vi "Save sxm File.vi"(4 "Parameters":string[][](array[string]), 5 "Auto file naming? (T)":bool=TRUE, 6 "Scanfield":T1, 7 "Scan param":T2, 8 "error in (no error)":errorcluster, 9 "Channels data":cluster{"Forward":sgl[][], "Backward":sgl[][]}[](array[cluster]), 10 "Channels config":T3(array[cluster]), 11 "Filename control":cluster{"Path":path, "Basename":string}={"Path"=path "C:/", "Basename"="unnamed"}) -> (0 "error out":errorcluster, 2 "File path out":path, 3 "Filename control out":cluster{"Path":path, "Basename":string}={"Path"=path "C:/", "Basename"="unnamed"})   [LabVIEW 2016, in "Nanonis Prog Interface.lvlib"]
doc: "<b>Saves a .sxm file.</b>\n\nIt saves the attributes in the header, and the channels configuration and their corresponding data into a .sxm file.\n\n<B>Auto file naming?</B>: if True (default), the file names are \"basenameNNN.sxm\" where NNN is an automatically increasing number.\n<B>Scan param</B>: scan direction Up (True) or Down (False), scan speed in seconds per line, start time, and end time.\n<B>Filename control</B>: the .sxm file is defined through a base path and a base name.\n<B>Channels config</B>: array of channels to save. Contains the channel name, calibration, offset, and channel index.\n<B>Channels data</B>: array of clusters containing forward and backward data for every channel.\n<B>Scanfield</B>: dimension of the scan field (center X & center Y, angle, width & height) and scan resolution (pixels & lines).\n<B>Parameters</B>: rest of header information. The first column should be filled in with the parameter name, and the second column with the parameter value.\nThe Bias value can be inserted using \"BIAS\" or \"Bias (V)\" as the parameter name. If no parameter with the latter name is found in the parameters array, then the file header will show a line as follows:\n:BIAS: n/a\n<B>File path out</B>: returns the full path of the saved fle.\n\nSeveral functions in the Scan palette (like ScanBuffer Get, ScanFrame Get, and Scan Grab Frame Data) can be used to feed in the required information from above.\n\n- Nanonis Programming Interface -"
uses:
  Nanonis Prog Interface.lvlib
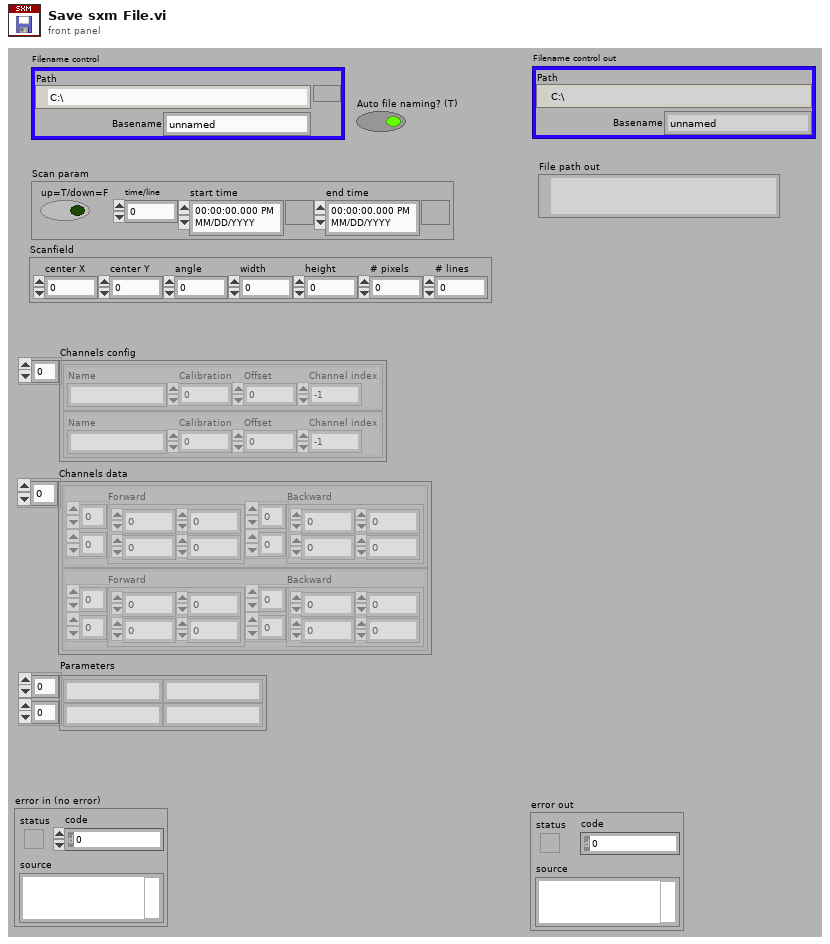
[diagram p1: front panel]
types:
  T1 = cluster{"center X":sgl, "center Y":sgl, "angle":sgl, "width":sgl, "height":sgl, "# pixels":i32, "# lines":i32}
  T2 = cluster{"up=T/down=F":bool, "time/line":sgl, "start time":timestamp, "end time":timestamp}
  T3 = cluster{"Name":string, "Calibration":sgl, "Offset":sgl, "Channel index":i32}[]
  T4 = enum16{"open", "replace", "create", "open or create", "replace or create", "replace or create with confirmation"}
  T5 = cluster{"Path":path, "Basename":string, "Extension":string}
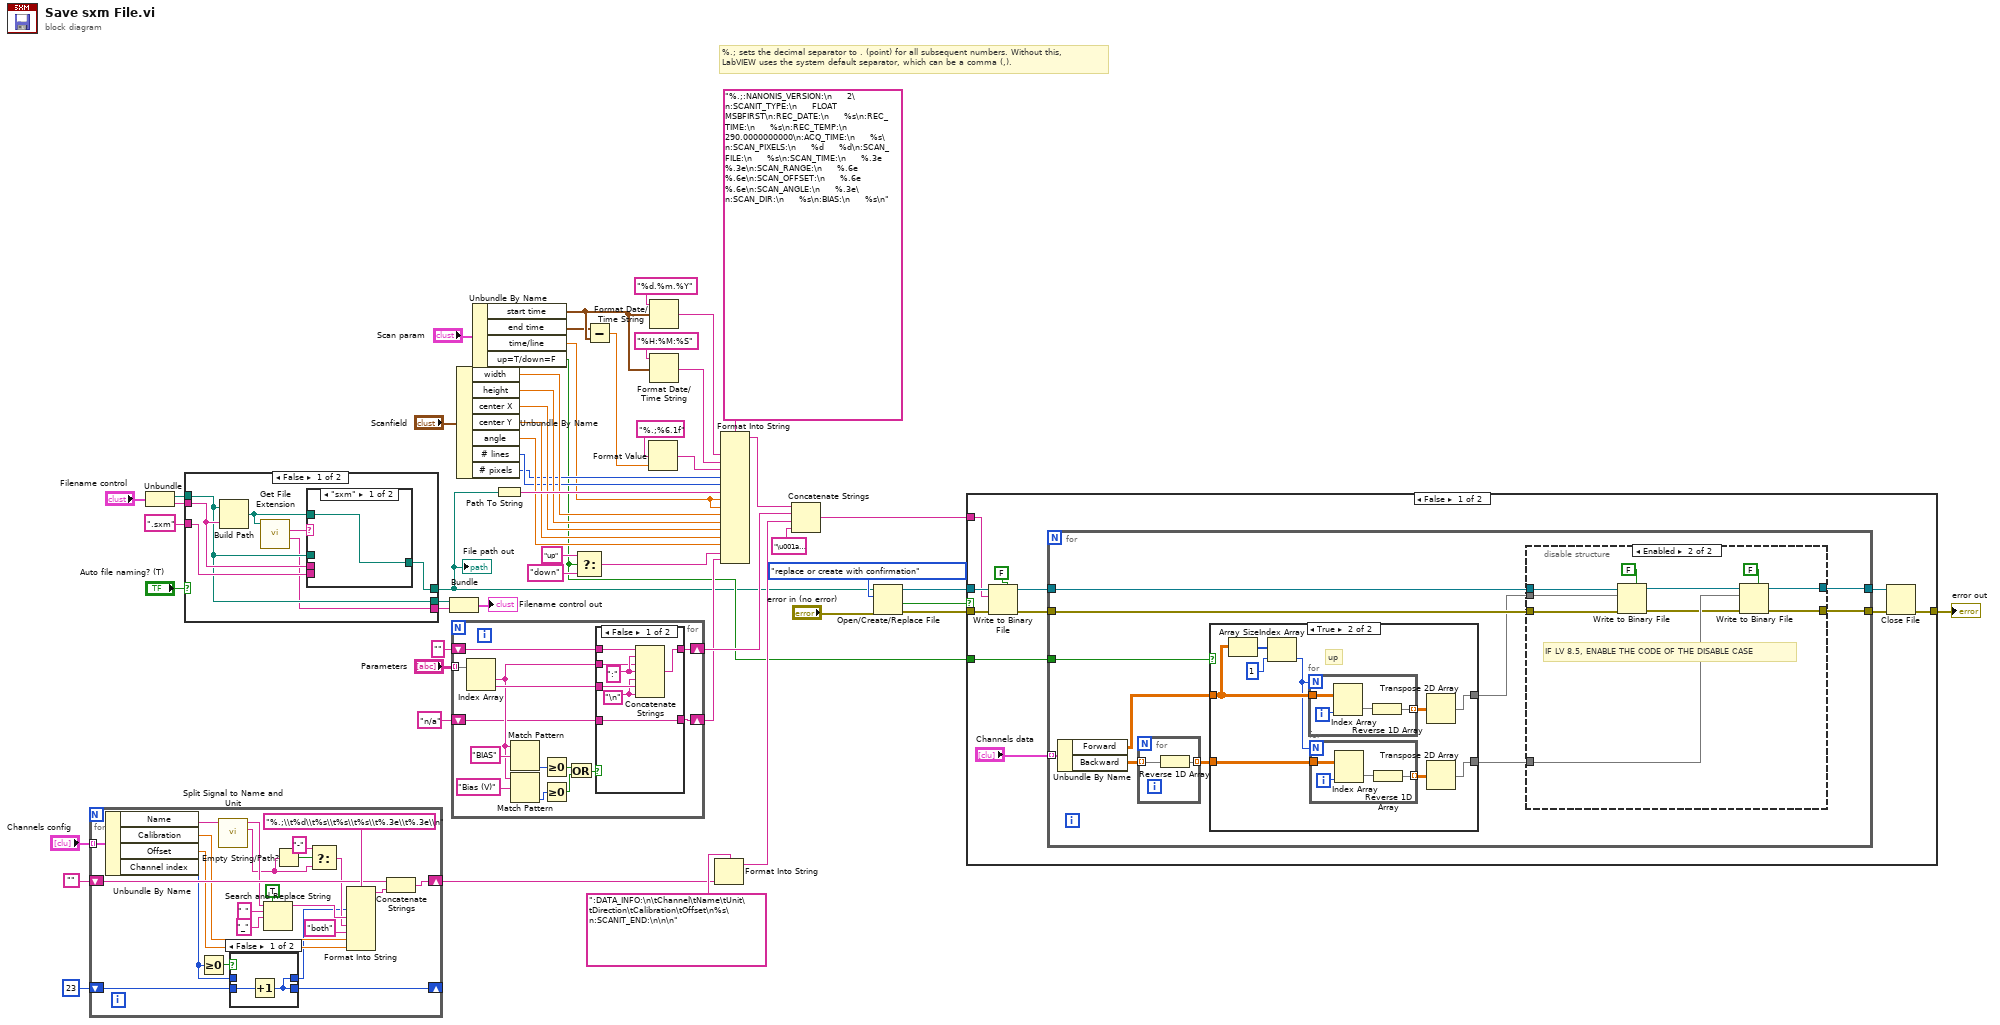
[diagram p0: block diagram]
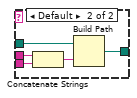
[diagram p3: hidden frame]
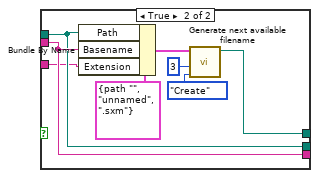
[diagram p4: hidden frame]
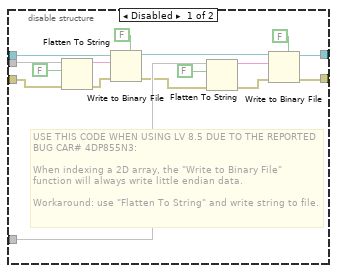
[diagram p5: hidden frame]
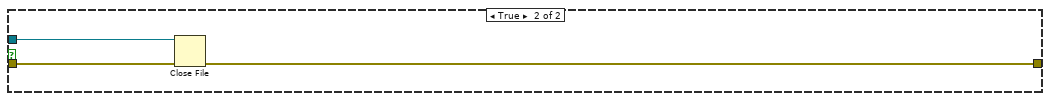
[diagram p7: hidden frame]
diagram:
  # "%.; sets the decimal separator to . (point) for all subsequent numbers. Without this, LabVIEW uses the system default separator, which can be a comma (,)."
  n1 = for {
    tunnel: "Channels config" -> [w77] mode=indexing
    shift-right: [w75] -> w39
    shift-left: "" -> [w74]
    shift-right: [w56] -> _
    shift-left: 23 -> [w57]
    n2 = Unbundle By Name(w77) -> ("Name"=w61:string, "Calibration"=w71:sgl, "Offset"=w70:sgl, "Channel index"=w60:i32)
    n3 = Greater Or Equal To 0?(x=w60) -> (x >= 0?=w58:bool)
    n4 = call <userlib>:"Split Signal to Name and Unit.vi"("Name with unit"=w61) -> ("Unit"=w55:string, "Name"=w66:string)  [unwired: 5 in]
    n5 = case shown="False" w58 {
      tunnel: w60 -> [_ w81]
      tunnel: [w78 w81] -> w59
      tunnel: w57 -> [w79 w80]
      tunnel: [w78 w80] -> w56
      frame False {
        n6 = Increment(x=w79) -> (x+1=w78:i32)
      }
      frame True {
      }
    }
    n7 = Search and Replace String(replace all?=TRUE ("replace all? (F)"), input string=w66, search string=" ", replace string="_" ("replace string (\"\")")) -> (result string=w67:string)  [unwired: 4 in, 3 out]
    n8 = Empty String/Path?(string/path=w55) -> (empty?=w64:bool)
    n9 = Select(t="-", s=w64, f=w55) -> (s? t:f=w63:string)
    n10 = Format Into String(format string="%.;\\t%d\\t%s\\t%s\\t%s\\t%.3e\\t%.3e\\n", w59, w67, w63, "both" ("input 4"), w71, w70) -> (resulting string=w73:string)  [unwired: 2 in, 1 out]
    n11 = Concatenate Strings(w74, w73) -> (w75:string)
  }
  n12 = Unbundle("Filename control") -> ("Path"=w15:path, "Basename"=w14:string)
  n13 = case shown="False" "Auto file naming? (T)" {
    tunnel: [w85 w100] -> w2
    tunnel: w15 -> [w83 w96]
    tunnel: w14 -> [w84 w97]
    tunnel: ".sxm" ("Extension") -> [w88 w95]
    tunnel: [w83 w96] -> w8
    tunnel: [w82 w97] -> w7
    frame False {
      n14 = Build Path(base path=w83, name or relative path=w84) -> (appended path=w86:path)
      n15 = call <vilib>:"Get File Extension.vi"("file"=w86) -> ("filename without extension"=w82:string, "lowercase file extension"=w87:string)  [unwired: 6 in, 3 out]
      n16 = case shown="\"sxm\"" w87 {
        tunnel: w88 -> [_ w94]
        tunnel: w86 -> [w89 _]
        tunnel: [w89 w90] -> w85
        tunnel: w83 -> [_ w92]
        tunnel: w84 -> [_ w91]
        frame "sxm" {
        }
        frame Default {
          n17 = Concatenate Strings(w91, w94) -> (w93:string)
          n18 = Build Path(base path=w92, name or relative path=w93) -> (appended path=w90:path)
        }
      }
    }
    frame True {
      n19 = Bundle By Name(cluster=T5 {"Path"=path "", "Basename"="unnamed", "Extension"=".sxm"} ("Filename control"), "Path"=w96, "Basename"=w97, "Extension"=w95) -> (w99:T5)
      n20 = call <userlib>:"Generate next available filename.vi"("Mode (Create)"=enum16{"Preview", "Create"}."Create", "Number of digits (3)"=u8 3, "Filename control"=w99) -> ("Next filename"=w100:path)  [unwired: 3 in, 1 out]
    }
  }
  "File path out" <- w2
  n21 = Bundle("Path"=w8, "Basename"=w7) -> (→"Filename control out":cluster{"Path":path, "Basename":string})  [unwired: 1 in]
  n22 = for {
    tunnel: "Parameters" -> [w116] mode=indexing
    shift-right: [w113] -> w5
    shift-left: "" ("format string") -> [w115]
    shift-right: [w104] -> w4
    shift-left: "n/a" ("f") -> [w103]
    n23 = Index Array(array=w116) -> (element #1=w110:string, element #2=w114:string)  [unwired: 2 in]
    n24 = Match Pattern(string=w110, regular expression="BIAS") -> (offset past match=w109:i32)  [unwired: 1 in, 3 out]
    n25 = Match Pattern(string=w110, regular expression="Bias (V)") -> (offset past match=w108:i32)  [unwired: 1 in, 3 out]
    n26 = Greater Or Equal To 0?(x=w109) -> (x >= 0?=w107:bool)
    n27 = Greater Or Equal To 0?(x=w108) -> (x >= 0?=w106:bool)
    n28 = Or(x=w107, y=w106) -> (x .or. y?=w105:bool)
    n29 = case shown="False" w105 {
      tunnel: w115 -> [w123 w125]
      tunnel: w114 -> [w121 w124]
      tunnel: [w120 w125] -> w113
      tunnel: w110 -> [w118 _]
      tunnel: [w117 w124] -> w104
      tunnel: w103 -> [w117 _]
      frame False {
        w119 = "\n" ("string")
        w122 = ":" ("string")
        n30 = Concatenate Strings(w123, w122, w118, w122, w119, w121, w119) -> (w120:string)
      }
      frame True {
      }
    }
  }
  n31 = Unbundle By Name("Scanfield") -> ("width"=w25:sgl, "height"=w24:sgl, "center X"=w23:sgl, "center Y"=w22:sgl, "angle"=w21:sgl, "# lines"=w20:i32, "# pixels"=w19:i32)
  n32 = Unbundle By Name("Scan param") -> ("start time"=w28:timestamp, "end time"=w27:timestamp, "time/line"=w18:sgl, "up=T/down=F"=w3:bool)
  n33 = Path To String(path=w2) -> (string=w52:string)
  n34 = Select(t="up", s=w3, f="down") -> (s? t:f=w42:string)
  n35 = Subtract(x=w27, y=w28) -> (x-y=w50:dbl)
  n36 = Format Value(format string="%.;%6.1f" ("time format string (%c)"), value (0)=w50) -> (output string=w51:string)  [unwired: 1 in]
  n37 = Format Date/Time String(time format string (%c)="%d.%m.%Y", seconds (now)=w28) -> (date/time string=w48:string)  [unwired: 1 in]
  n38 = Format Date/Time String(time format string (%c)="%H:%M:%S", seconds (now)=w28) -> (date/time string=w49:string)  [unwired: 1 in]
  n39 = Format Into String(format string=":DATA_INFO:\n\tChannel\tName\tUnit\tDirection\tCalibration\tOffset\n%s\n:SCANIT_END:\n\n\n", w39) -> (resulting string=w11:string)  [unwired: 2 in, 1 out]
  n40 = Format Into String(format string="%.;:NANONIS_VERSION:\n     2\n:SCANIT_TYPE:\n     FLOAT     MSBFIRST\n:REC_DATE:\n     %s\n:REC_TIME:\n     %s\n:REC_TEMP:\n     290.0000000000\n:ACQ_TIME:\n     %s\n:SCAN_PIXELS:\n     %d     %d\n:SCAN_FILE:\n     %s\n:SCAN_TIME:\n     %.3e     %.3e\n:SCAN_RANGE:\n     %.6e     %.6e\n:SCAN_OFFSET:\n     %.6e     %.6e\n:SCAN_ANGLE:\n     %.3e\n:SCAN_DIR:\n     %s\n:BIAS:\n     %s\n", w48, w49, w51, w19, w20, w52, w18, w18, w25, w24, w23, w22, w21, w42, w4) -> (resulting string=w33:string)  [unwired: 2 in, 1 out]
  n41 = Concatenate Strings(w33, w5, w11, "\u001a\u0004" ("string")) -> (w36:string)
  n42 = Open/Create/Replace File(file path (use dialog)=w2, error in="error in (no error)", operation (0:open)=T4."replace or create with confirmation") -> (refnum out=w37:refnum<file>, cancelled=w32:bool, error out=w35:errorcluster)  [unwired: 3 in]
  n43 = case shown="False" w32 {
    tunnel: [w129 w195] -> w31
    tunnel: w37 -> [w135 w197]
    tunnel: w36 -> [w134 _]
    tunnel: w35 -> [w133 w196]
    tunnel: w3 -> [w126 _]
    frame False {
      n44 = Write to Binary File(file (use dialog)=w135, data=w134, error in=w133, 5:FALSE ("prepend array or string size? (T)")) -> (refnum out=w131:refnum<file>, error out=w132:errorcluster)  [unwired: 2 in, 1 out]
      n45 = for {
        tunnel: w132 -> [w141]
        tunnel: w131 -> [w142]
        tunnel: [w140] -> w130
        tunnel: [w139] -> w128
        tunnel: "Channels data" -> [w147] mode=indexing
        tunnel: w126 -> [w145]
        n46 = Unbundle By Name(w147) -> ("Forward"=w146:sgl[][], "Backward"=w144:sgl[][])
        n47 = for {
          tunnel: w144 -> [w194] mode=indexing
          tunnel: [w193] -> w143 mode=indexing
          n48 = Reverse 1D Array(array=w194) -> (reversed array=w193:sgl[])
        }
        n49 = case shown="True" w145 {
          tunnel: w143 -> [w174 w176]
          tunnel: [w174 w177] -> w138
          tunnel: w146 -> [w175 w182]
          tunnel: [w175 w181] -> w137
          frame False {
            # "down"
          }
          frame True {
            # "up"
            n50 = Array Size(array=w182) -> (size(s)=w183:i32[])
            n51 = Index Array(array=w183, index=1) -> (element=w178:i32)
            n52 = for {
              N: w178 -> [_]
              tunnel: w182 -> [w192]
              tunnel: [w189] -> w184 mode=indexing
              i -> [w191]
              n53 = Index Array(array=w192, index (col)=w191) -> (element=w190:sgl[])  [unwired: 1 in]
              n54 = Reverse 1D Array(array=w190) -> (reversed array=w189:sgl[])
            }
            n55 = for {
              N: w178 -> [_]
              tunnel: w176 -> [w188]
              tunnel: [w185] -> w179 mode=indexing
              i -> [w187]
              n56 = Index Array(array=w188, index (col)=w187) -> (element=w186:sgl[])  [unwired: 1 in]
              n57 = Reverse 1D Array(array=w186) -> (reversed array=w185:sgl[])
            }
            n58 = Transpose 2D Array(2D array=w184) -> (transposed array=w181:sgl[][])
            n59 = Transpose 2D Array(2D array=w179) -> (transposed array=w177:sgl[][])
          }
        }
        n60 = disable-structure shown="Enabled" {
          disable-tunnel: w137 -> [w163 w170]
          disable-tunnel: w138 -> [w153 w169]
          disable-tunnel: w142 -> [w156 w167]
          disable-tunnel: w141 -> [w151 w166]
          disable-tunnel: [w154 w165] -> w139
          disable-tunnel: [w152 w164] -> w140
          frame Disabled {
            # "USE THIS CODE WHEN USING LV 8.5 DUE TO THE REPORTED BUG CAR# 4DP855N3:\n\nWhen indexing a 2D array, the \"Write to Binary File\" function will always write little endian data.\n\nWorkaround: use \"Flatten To String\" and write string to file."
            n61 = Flatten To String(anything=w163, prepend array or string size? (T)=FALSE, error in (no error)=w151) -> (data string=w160:string, error out=w150:errorcluster)  [unwired: 1 in, 1 out]
            n62 = Write to Binary File(file (use dialog)=w156, data=w160, error in=w150, 5:FALSE ("prepend array or string size? (T)")) -> (refnum out=w155:refnum<file>, error out=w149:errorcluster)  [unwired: 2 in, 1 out]
            n63 = Flatten To String(anything=w153, prepend array or string size? (T)=FALSE, error in (no error)=w149) -> (data string=w159:string, error out=w148:errorcluster)  [unwired: 1 in, 1 out]
            n64 = Write to Binary File(file (use dialog)=w155, data=w159, error in=w148, 5:FALSE ("prepend array or string size? (T)")) -> (refnum out=w154:refnum<file>, error out=w152:errorcluster)  [unwired: 2 in, 1 out]
          }
          frame Enabled {
            # "IF LV 8.5, ENABLE THE CODE OF THE DISABLE CASE"
            n65 = Write to Binary File(file (use dialog)=w167, data=w170, error in=w166, 5:FALSE ("prepend array or string size? (T)")) -> (refnum out=w171:refnum<file>, error out=w168:errorcluster)  [unwired: 2 in, 1 out]
            n66 = Write to Binary File(file (use dialog)=w171, data=w169, error in=w168, 5:FALSE ("prepend array or string size? (T)")) -> (refnum out=w165:refnum<file>, error out=w164:errorcluster)  [unwired: 2 in, 1 out]
          }
        }
      }
      n67 = Close File(refnum=w128, error in=w130) -> (error out=w129:errorcluster)  [unwired: 1 out]
    }
    frame True {
      n68 = Close File(refnum=w197, error in=w196) -> (error out=w195:errorcluster)  [unwired: 1 out]
    }
  }
  "error out" <- w31
